vi "Set Output Channel.vi"(0 "Scaling configuration in":refnum<class "Scaling configuration.lvclass">, 5 "Channel":refnum<class "TBM channel.lvclass">, 7 "Scale Index":i32, 9 "Mapping Index":i32, 11 "error in (no error)":errorcluster) -> (4 "Scaling configuration out":refnum<class "Scaling configuration.lvclass">, 15 "error out":errorcluster)   [LabVIEW 2013, in "Scaling configuration.lvclass"]
uses:
  Scaling configuration.lvclass
  <vilib>/NI/Tag Bus Module Framework/channel/TBM channel.lvclass
  Scaling configuration.lvclass/Scaling configuration.ctl
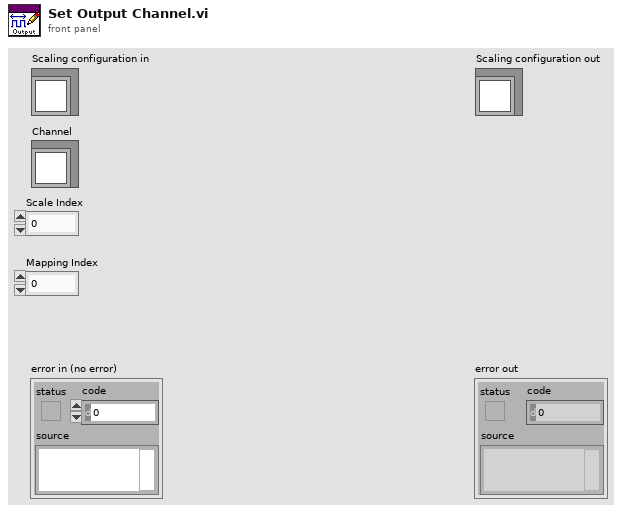
[diagram p1: front panel]
types:
  T1 = typedef "Scaling configuration.lvclass/scale data types.ctl" = enum16{"Double", "Single", "I64", "I32", "I16", "I8", "U64", "U32", "U16", "U8"}
  T2 = cluster{"mappings":cluster{"input channel":refnum<class "TBM channel.lvclass">, "output channel":refnum<class "TBM channel.lvclass">, "input data type":T1, "output data type":T1}[], "name":string}[]
  T3 = cluster{"mappings":cluster{"input channel":refnum<class "TBM channel.lvclass">, "output channel":refnum<class "TBM channel.lvclass">, "input data type":T1, "output data type":T1}[], "name":string}
  T4 = cluster{"input channel":refnum<class "TBM channel.lvclass">, "output channel":refnum<class "TBM channel.lvclass">, "input data type":T1, "output data type":T1}[]
  T5 = cluster{"input channel":refnum<class "TBM channel.lvclass">, "output channel":refnum<class "TBM channel.lvclass">, "input data type":T1, "output data type":T1}
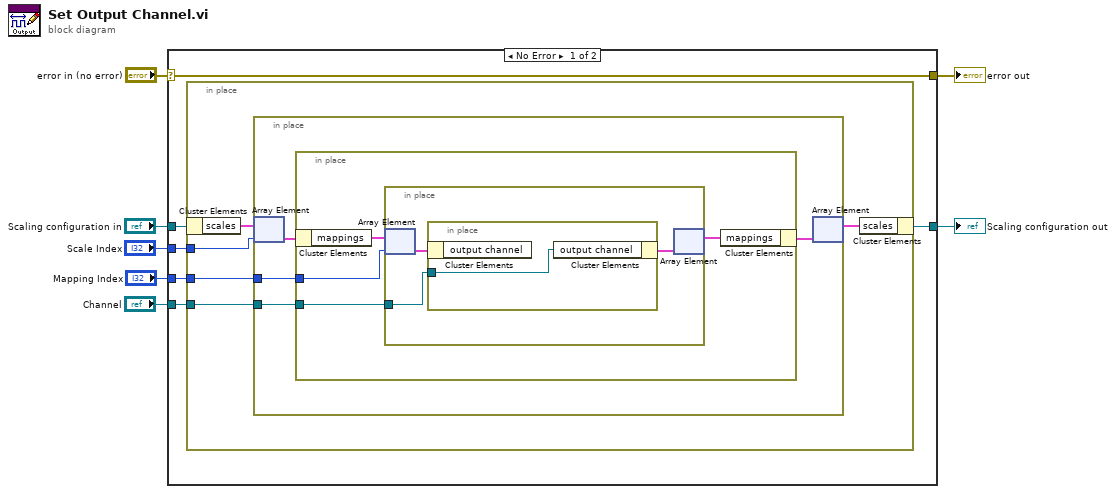
[diagram p0: block diagram]
diagram:
  n1 = case shown="No Error" "error in (no error)" {
    selector: "error in (no error)" -> [w13 w32]
    tunnel: [w13 w32] -> w6
    tunnel: [w10 w31] -> w4
    tunnel: "Scaling configuration in" -> [w12 w31]
    tunnel: "Scale Index" -> [w11 _]
    tunnel: "Mapping Index" -> [w9 _]
    tunnel: "Channel" -> [w8 _]
    frame No Error {
      n2 = in-place {
        in-place-border: w11 -> [w17]
        in-place-border: w9 -> [w15]
        in-place-border: w8 -> [w14]
        n3 = in-place-cluster #1(w12) -> ("scales"=w18:T2)
        n4 = in-place {
          in-place-border: w15 -> [w20]
          in-place-border: w14 -> [w19]
          n5 = in-place-array #2(w18, w17) -> (w22:T3)
          n6 = in-place {
            in-place-border: w20 -> [w24]
            in-place-border: w19 -> [w23]
            n7 = in-place-cluster #3(w22) -> ("mappings"=w26:T4)
            n8 = in-place {
              in-place-border: w23 -> [w28]
              n9 = in-place-array #4(w26, w24) -> (w29:T5)
              n10 = in-place {
                in-place-border: w28 -> [w30]
                n11 = in-place-cluster #5(w29) -> ()  [unwired: 1 out]
                n12 = in-place-cluster #5("output channel"=w30) -> (w27:T5)
              }
              n13 = in-place-array #4(w27) -> (w25:T4)  [unwired: 1 out]
            }
            n14 = in-place-cluster #3("mappings"=w25) -> (w21:T3)
          }
          n15 = in-place-array #2(w21) -> (w16:T2)  [unwired: 1 out]
        }
        n16 = in-place-cluster #1("scales"=w16) -> (w10:refnum<class "Scaling configuration.lvclass">)
      }
    }
    frame Error {
    }
  }
  "error out" <- w6
  "Scaling configuration out" <- w4
